vi "add vision spectrum.vi"(0 "display array in":T1(array[cluster]), 1 "number of gated regions":i32, 9 "channel 0-4 energy out":u32[][](array[numeric]), 11 "error in (no error)":errorcluster, 12 "pulses recieved":u32, 14 "labview time":dbl) -> (3 "run time":dbl, 4 "display array out":T1(array[cluster]), 5 "rare count per iteration":dbl, 6 "rare count rate(cps)":dbl, 10 "live time(%)":dbl, 13 "total rare counts":dbl, 15 "error out":errorcluster)   [LabVIEW 2016]
doc: "Takes the new spill of data from the pixie and adds it to the number of spectrum that is being used"
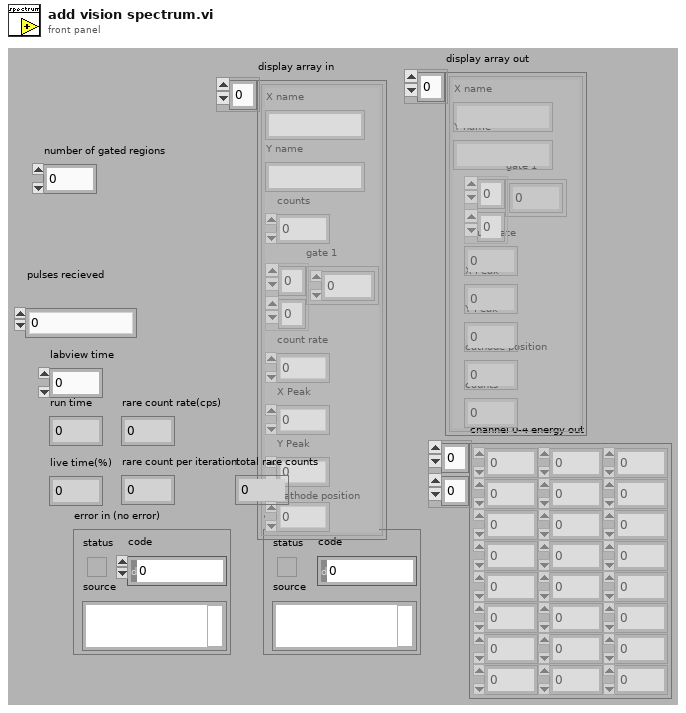
[diagram p1: front panel]
types:
  T1 = cluster{"X name":string, "Y name ":string, "counts":dbl, "gate 1":dbl[][], "count rate":dbl, "X Peak":dbl, "Y Peak":dbl, "cathode position":dbl}[]
  T2 = cluster{"X name":string, "Y name ":string, "counts":dbl, "gate 1":dbl[][], "count rate":dbl, "stable 1":dbl, "stable 2":dbl, "cathode position":dbl}[]
  T3 = cluster{"X name":string, "Y name ":string, "counts":dbl, "gate 1":dbl[][], "count rate":dbl, "X Peak":dbl, "Y Peak":dbl, "cathode position":dbl}
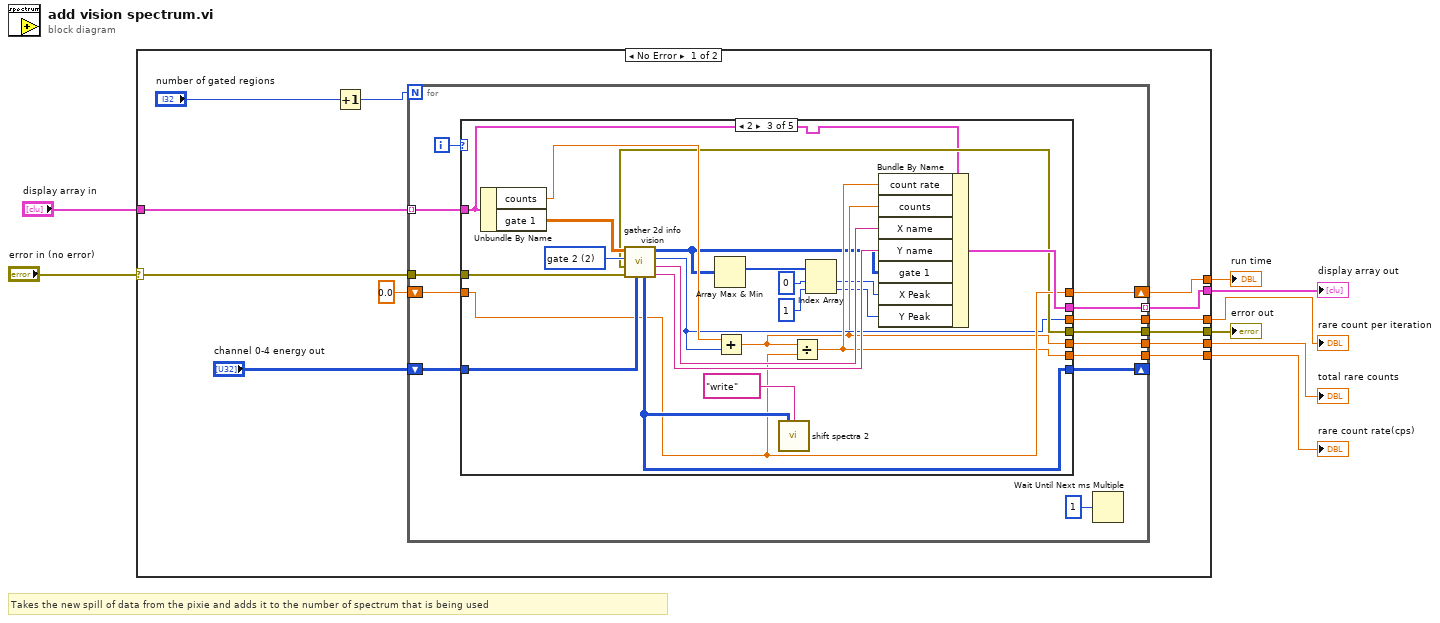
[diagram p0: block diagram]
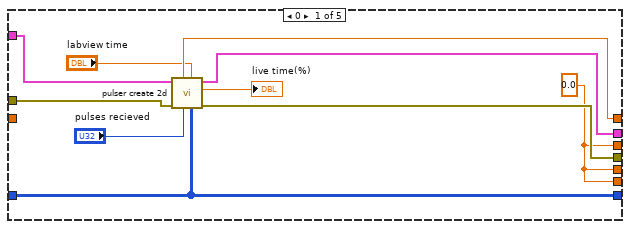
[diagram p2: hidden frame]
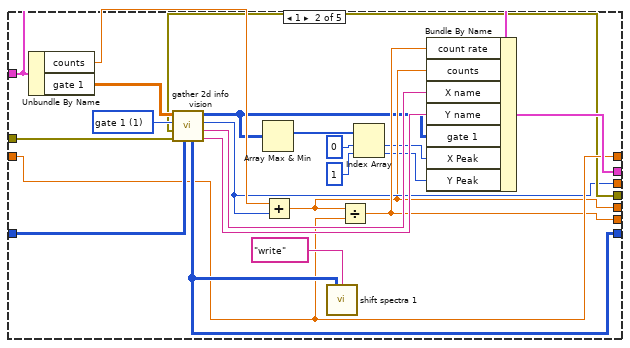
[diagram p3: hidden frame]
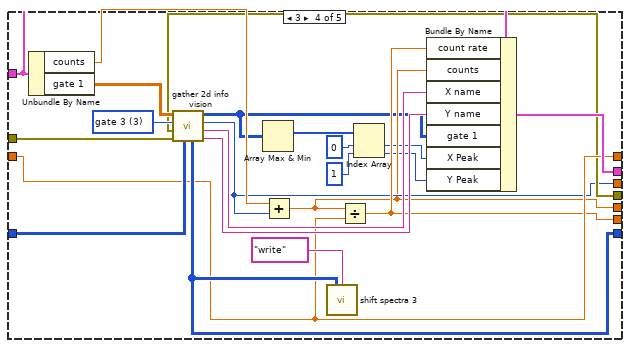
[diagram p4: hidden frame]
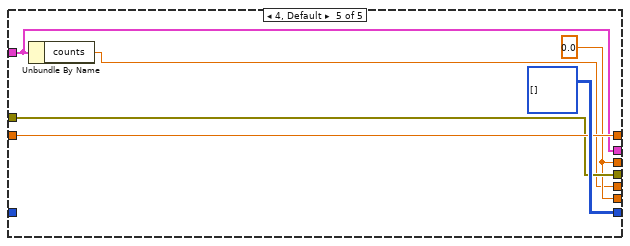
[diagram p5: hidden frame]
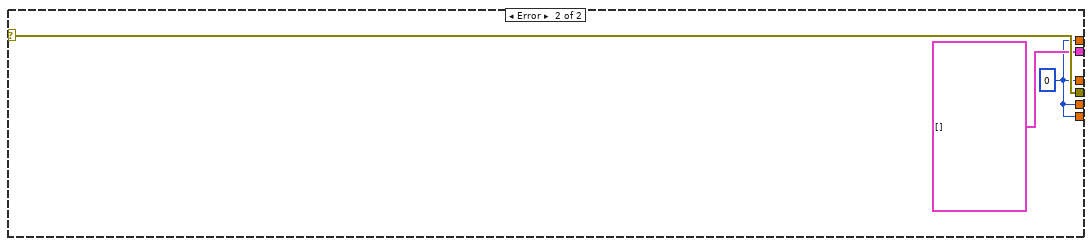
[diagram p6: hidden frame]
diagram:
  # "Takes the new spill of data from the pixie and adds it to the number of spectrum that is being used"
  n1 = case shown="No Error" "error in (no error)" {
    selector: "error in (no error)" -> [w15 w118]
    tunnel: [w14 w118] -> w7
    tunnel: [w16 w116] -> w6
    tunnel: [w13 w116] -> w5
    tunnel: [w12 T2 [] ("display array out 2")] -> w4
    tunnel: [w11 w116] -> w3
    tunnel: [w10 w116] -> w2
    tunnel: "display array in" -> [w9 _]
    frame No Error {
      n2 = Increment(x="number of gated regions") -> (x+1=w20:i32)
      n3 = for {
        N: w20 -> [_]
        shift-right: [w33] -> _
        shift-left: "channel 0-4 energy out" -> [w32]
        tunnel: [w30] -> w12 mode=indexing
        tunnel: w9 -> [w29] mode=indexing
        shift-right: [w28] -> w16
        shift-left: 0.0 -> [w27]
        tunnel: w15 -> [w26]
        tunnel: [w25] -> w14
        tunnel: [w24] -> w13
        tunnel: [w22] -> w11
        tunnel: [w21] -> w10
        i -> [w31]
        n4 = case shown="2" w31 {
          tunnel: [w43 w62 w85 w107 u32[][] [] ("intensity array out")] -> w33
          tunnel: w32 -> [w43 w63 w86 w108 _]
          tunnel: w29 -> [w35 w57 w66 w101 w111]
          tunnel: [w42 w61 w83 w105 w111] -> w30
          tunnel: [w40 w55 w78 w99 w114] -> w28
          tunnel: w27 -> [_ w55 w78 w99 w114]
          tunnel: w26 -> [w39 w54 w76 w97 w113]
          tunnel: [w38 w53 w77 w98 w113] -> w25
          tunnel: [w34 w52 w75 w96 w112] -> w24
          tunnel: [w34 w51 w74 w95 w112] -> w22
          tunnel: [w34 w50 w73 w94 w110] -> w21
          frame 0 {
            w34 = 0.0
            n5 = call "pulser create 2d.vi"("channel 0-4 energy in"=w43, "labview time"="labview time", "pulses recieved"="pulses recieved", "error in (no error)"=w39, "xy position cluster"=w35) -> ("error out"=w38:errorcluster, "live time(%)"=→"live time(%)":dbl, "xy position cluster out"=w42:T3, "run time"=w40:dbl)  [unwired: 3 in]
          }
          frame 1 {
            w64 = u16 1 items=["pulser", "gate 1", "gate 2", "gate 3", "none"] ("which gate")
            n6 = Unbundle By Name(w57) -> ("counts"=w58:dbl, "gate 1"=w56:dbl[][])
            n7 = call "gather 2d info vision.vi"("channel 0-4 energy in"=w63, "error in (no error)"=w54, "which gate"=w64, "New Image"=w56) -> ("Y name output"=w59:string, "X name output"=w60:string, "sum of counts out"=w51:i32, "New Image out"=w49:i32[][], "Peak height out"=w62:i32[][], "error out"=w53:errorcluster)  [unwired: 1 in, 1 out]
            n8 = Array Max & Min(array=w49) -> (max index (indices)=w48:i32[])  [unwired: 3 out]
            n9 = Add(x=w58, y=w51) -> (x+y=w50:dbl)
            n10 = call "shift spectra 1.vi"("2d intensity array"=w62, "shift control"="write") -> ()  [unwired: 7 in, 7 out]
            n11 = Divide(x=w50, y=w55) -> (x/y=w52:dbl)
            n12 = Index Array(array=w48, index #1=0 ("index"), index #2=1 ("index")) -> (element #1=w44:i32, element #2=w45:i32)
            n13 = Bundle By Name(cluster=w57, "count rate"=w52, "counts"=w50, "X name"=w60, "Y name"=w59, "gate 1"=w49, "X Peak"=w44, "Y Peak"=w45) -> (w61:T3)
          }
          frame 2 {
            w84 = u16 2 items=["pulser", "gate 1", "gate 2", "gate 3", "none"] ("which gate")
            n14 = Unbundle By Name(w66) -> ("counts"=w80:dbl, "gate 1"=w79:dbl[][])
            n15 = call "gather 2d info vision.vi"("channel 0-4 energy in"=w86, "error in (no error)"=w76, "which gate"=w84, "New Image"=w79) -> ("Y name output"=w81:string, "X name output"=w82:string, "sum of counts out"=w74:i32, "New Image out"=w69:i32[][], "Peak height out"=w85:i32[][], "error out"=w77:errorcluster)  [unwired: 1 in, 1 out]
            n16 = Array Max & Min(array=w69) -> (max index (indices)=w72:i32[])  [unwired: 3 out]
            n17 = Add(x=w80, y=w74) -> (x+y=w73:dbl)
            n18 = call "shift spectra 2.vi"("2d intensity array"=w85, "shift control"="write") -> ()  [unwired: 7 in, 7 out]
            n19 = Divide(x=w73, y=w78) -> (x/y=w75:dbl)
            n20 = Index Array(array=w72, index #1=0 ("index"), index #2=1 ("index")) -> (element #1=w68:i32, element #2=w67:i32)
            n21 = Bundle By Name(cluster=w66, "count rate"=w75, "counts"=w73, "X name"=w82, "Y name"=w81, "gate 1"=w69, "X Peak"=w68, "Y Peak"=w67) -> (w83:T3)
          }
          frame 3 {
            w106 = u16 3 items=["pulser", "gate 1", "gate 2", "gate 3", "none"] ("which gate")
            n22 = Unbundle By Name(w101) -> ("counts"=w102:dbl, "gate 1"=w100:dbl[][])
            n23 = call "gather 2d info vision.vi"("channel 0-4 energy in"=w108, "error in (no error)"=w97, "which gate"=w106, "New Image"=w100) -> ("Y name output"=w103:string, "X name output"=w104:string, "sum of counts out"=w95:i32, "New Image out"=w90:i32[][], "Peak height out"=w107:i32[][], "error out"=w98:errorcluster)  [unwired: 1 in, 1 out]
            n24 = Array Max & Min(array=w90) -> (max index (indices)=w93:i32[])  [unwired: 3 out]
            n25 = Add(x=w102, y=w95) -> (x+y=w94:dbl)
            n26 = call "shift spectra 3.vi"("2d intensity array"=w107, "shift control"="write") -> ()  [unwired: 7 in, 7 out]
            n27 = Divide(x=w94, y=w99) -> (x/y=w96:dbl)
            n28 = Index Array(array=w93, index #1=0 ("index"), index #2=1 ("index")) -> (element #1=w89:i32, element #2=w88:i32)
            n29 = Bundle By Name(cluster=w101, "count rate"=w96, "counts"=w94, "X name"=w104, "Y name"=w103, "gate 1"=w90, "X Peak"=w89, "Y Peak"=w88) -> (w105:T3)
          }
          frame 4, Default {
            w112 = 0.0
            n30 = Unbundle By Name(w111) -> ("counts"=w110:dbl)
          }
        }
        n31 = Wait Until Next ms Multiple(millisecond multiple=u32 1) -> ()  [unwired: 1 out]
      }
    }
    frame Error {
      w116 = 0 ("sum of counts out")
    }
  }
  "error out" <- w7
  "run time" <- w6
  "rare count rate(cps)" <- w5
  "display array out" <- w4
  "rare count per iteration" <- w3
  "total rare counts" <- w2
